vi "Update_Functions.vi"(2 "Debug":bool, 3 "API Function Array":cluster{string, "VI Reference":refnum<vi>}[](array[cluster]), 4 "Event":cluster{string, string[], dbl[], dbl}, 5 "Update Functions In":cluster{string, string[], dbl[], dbl}[](array[cluster])) -> (0 "Status Array":cluster{string[], "Status Out":string}[](array[cluster]), 1 "Update Functions Out":cluster{string, string[], dbl[], dbl}[](array[cluster]))   [LabVIEW 2011]
doc: "This VI examines a new event given by the \"Event\" parameter, and if necessary, adds or removes the appropriate functions from the \"Update Functions\" array. \"Debug\" disables all external hardware communications."
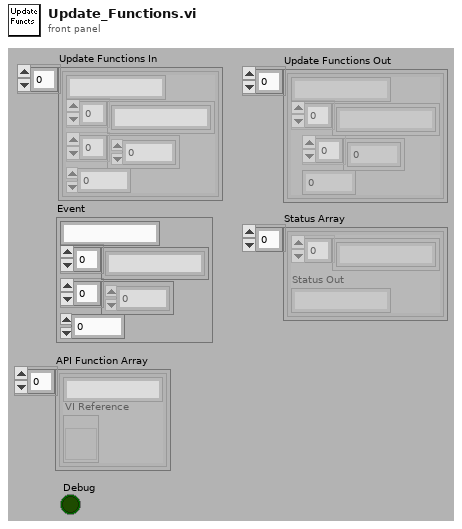
[diagram p1: front panel]
types:
  T1 = enum16{"Discrete", "Continuous", "Instantaneous", "Finite"}
  T2 = cluster{string, "Argument List Out":string[], dbl[], "element":dbl}
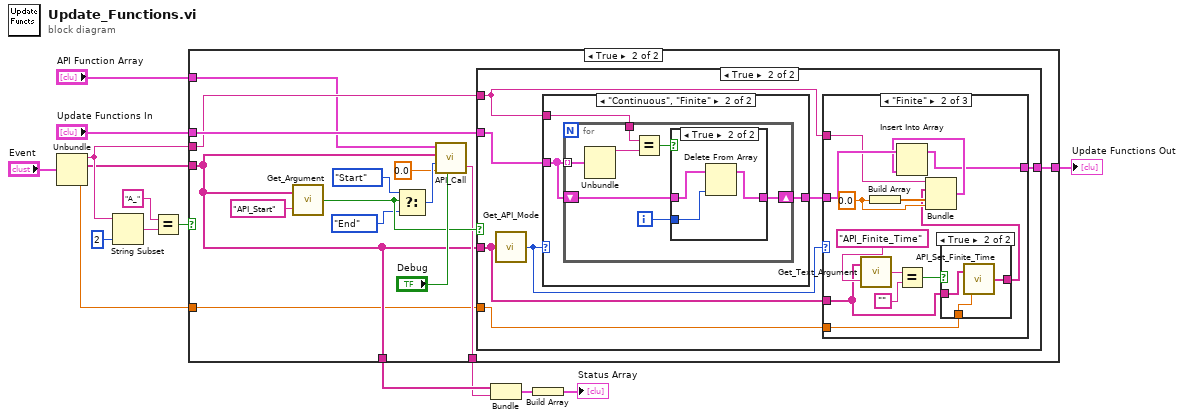
[diagram p0: block diagram]
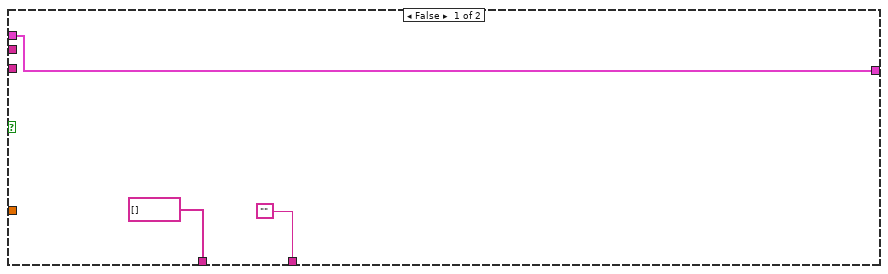
[diagram p2: hidden frame]
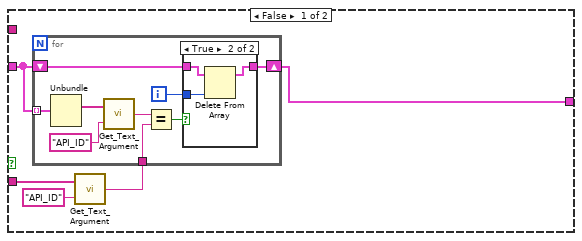
[diagram p3: hidden frame]
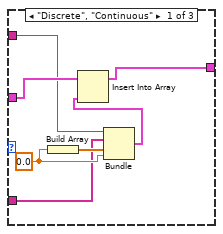
[diagram p5: hidden frame]
diagram:
  n1 = Unbundle("Event") -> (w10:string, w6:string[], w1:dbl)  [unwired: 1 out]
  n2 = String Subset(string=w10, length (rest)=2 ("length (rest)")) -> (substring=w12:string)  [unwired: 1 out]
  n3 = Equal?(x="A_" ("substring"), y=w12) -> (x = y?=w11:bool)
  n4 = case shown="True" w11 {
    tunnel: "Update Functions In" -> [w18 w32]
    tunnel: w10 -> [_ w31]
    tunnel: w6 -> [_ w20]
    tunnel: [w18 w24] -> w8
    tunnel: "API Function Array" -> [_ w23]
    tunnel: ["" w21] -> w4
    tunnel: [string[] [] w20] -> w5
    tunnel: w1 -> [_ w19]
    frame False {
    }
    frame True {
      n5 = call "Get_Argument.vi"("Argument"="API_Start", "Argument List"=w20) -> ("Enabled"=w27:bool)
      n6 = Select(t=enum16{"Edit", "Start", "Run", "End", "Idle"}."Start" ("State"), s=w27, f=enum16{"Edit", "Start", "Run", "End", "Idle"}."End" ("State")) -> (s? t:f=w28:enum16{"Edit", "Start", "Run", "End", "Idle"})
      n7 = call "API_Call.vi"("API Function Array"=w23, "Argument List In"=w20, "State"=w28, "Elapsed Time (s)"=0.0, "Debug Mode"="Debug") -> ("Status Out"=w21:string)  [unwired: 1 out]
      n8 = case shown="True" w27 {
        tunnel: w31 -> [_ w54]
        tunnel: w32 -> [w35 w57]
        tunnel: w20 -> [w37 w51]
        tunnel: [w33 w53] -> w24
        tunnel: w19 -> [_ w52]
        frame False {
          n9 = call "Get_Text_Argument.vi"("Argument"="API_ID", "Argument List"=w37) -> ("Text"=w34:string)
          n10 = for {
            tunnel: w35 -> [w46] mode=indexing
            shift-right: [w38] -> w33
            shift-left: w35 -> [w40]
            tunnel: w34 -> [w42]
            i -> [w39]
            n11 = Unbundle(w46) -> (w45:string[])  [unwired: 3 out]
            n12 = call "Get_Text_Argument.vi"("Argument"="API_ID", "Argument List"=w45) -> ("Text"=w43:string)
            n13 = Equal?(x=w43, y=w42) -> (x = y?=w41:bool)
            n14 = case shown="True" w41 {
              tunnel: w40 -> [w47 w50]
              tunnel: w39 -> [_ w49]
              tunnel: [w47 w48] -> w38
              frame False {
              }
              frame True {
                n15 = Delete From Array(array=w50, index=w49) -> (array with subset deleted=w48:cluster{string, string[], dbl[], dbl}[])  [unwired: 1 in, 1 out]
              }
            }
          }
        }
        frame True {
          n16 = call "Get_API_Mode.vi"("Argument List"=w51) -> ("API Mode"=w56:T1)
          n17 = case shown="\"Continuous\", \"Finite\"" w56 {
            tunnel: w57 -> [w83 w85]
            tunnel: w54 -> [_ w86]
            tunnel: [w83 w84] -> w55
            frame Default {
            }
            frame "Continuous", "Finite" {
              n18 = for {
                tunnel: w85 -> [w93] mode=indexing
                tunnel: w86 -> [w92]
                shift-right: [w87] -> w84
                shift-left: w85 -> [w89]
                i -> [w88]
                n19 = Unbundle(w93) -> (w91:string)  [unwired: 3 out]
                n20 = Equal?(x=w92, y=w91) -> (x = y?=w90:bool)
                n21 = case shown="True" w90 {
                  tunnel: w89 -> [w94 w97]
                  tunnel: w88 -> [_ w96]
                  tunnel: [w94 w95] -> w87
                  frame False {
                  }
                  frame True {
                    n22 = Delete From Array(array=w97, index=w96) -> (array with subset deleted=w95:cluster{string, string[], dbl[], dbl}[])  [unwired: 1 in, 1 out]
                  }
                }
              }
            }
          }
          n23 = case shown="\"Finite\"" w56 {
            tunnel: w55 -> [w64 w77 w82]
            tunnel: w54 -> [w63 w76 _]
            tunnel: [w59 w72 w82] -> w53
            tunnel: w52 -> [_ w66 _]
            tunnel: w51 -> [w58 w67 _]
            frame "Discrete", "Continuous" {
              w61 = 0.0 ("element")
              n24 = Build Array(w61) -> (w62:dbl[])
              n25 = Bundle(w63, w58, w62, "element"=w61) -> (w60:cluster{string, string[], dbl[], "element":dbl})  [unwired: 1 out]
              n26 = Insert Into Array(array=w64, new element=w60) -> (w59:cluster{string, string[], dbl[], dbl}[])  [unwired: 1 in]
            }
            frame "Finite" {
              w74 = 0.0 ("element")
              n27 = call "Get_Text_Argument.vi"("Argument"="API_Finite_Time", "Argument List"=w67) -> ("Text"=w70:string)
              n28 = Build Array(w74) -> (w75:dbl[])
              n29 = Equal?(x=w70, y="") -> (x = y?=w68:bool)
              n30 = case shown="True" w68 {
                tunnel: w67 -> [w78 w81]
                tunnel: w66 -> [_ w80]
                tunnel: [w78 w79] -> w65
                frame False {
                }
                frame True {
                  n31 = call "API_Set_Finite_Time.vi"("Finite Time"=w80, "Argument List In"=w81) -> ("Argument List Out"=w79:string[])
                }
              }
              n32 = Bundle(w76, "Argument List Out"=w65, w75, "element"=w74) -> (w73:T2)  [unwired: 1 out]
              n33 = Insert Into Array(array=w77, new element=w73) -> (w72:cluster{string, string[], dbl[], dbl}[])  [unwired: 1 in]
            }
            frame "Instantaneous", Default {
            }
          }
        }
      }
    }
  }
  "Update Functions Out" <- w8
  n34 = Bundle(w5, "Status Out"=w4) -> (w3:cluster{string[], "Status Out":string})  [unwired: 1 in]
  n35 = Build Array(w3) -> (→"Status Array":cluster{string[], "Status Out":string}[])
